vi "testSharedVariable.vi"() -> ()   [LabVIEW 2015]
uses:
  state.ctl
  MyToolsStatus.lvlib
panel:
  in  "Cluster":T1
  out "error out":errorcluster
  in  "stop":bool
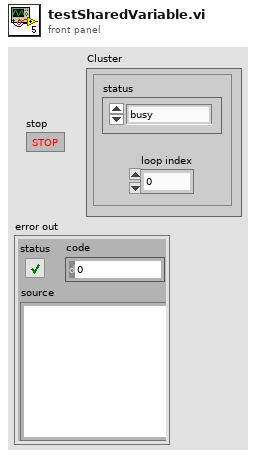
[diagram p1: front panel]
types:
  T1 = typedef "MyToolsStatus.lvlib/state.ctl" = cluster{"loop index":i32, "status":enum16{"busy", "ready", "error"}}
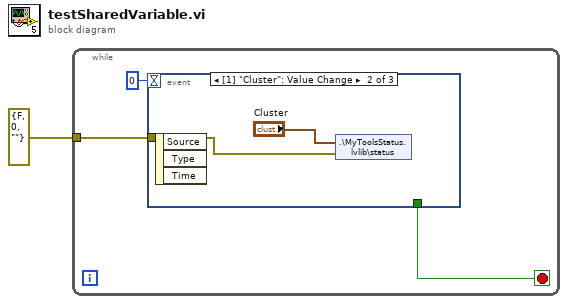
[diagram p0: block diagram]
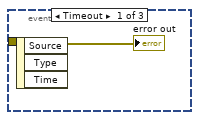
[diagram p2: hidden frame]
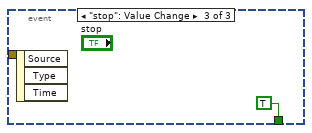
[diagram p3: hidden frame]
diagram:
  n1 = while {
    tunnel: errorcluster {"status"=FALSE, "code"=0, "source"=""} ("error in (no error)") -> [w4]
    stop <- w3 stop-if-true
    n2 = event shown="[1] \"Cluster\": Value Change" {
      selector: _ -> [_ _ _]
      dyn-events: _ -> [_ _ _]
      timeout: 0 -> [_ _ _]
      tunnel: w4 -> [w5 w7 _]
      tunnel: [_ _ TRUE] -> w3
      event Timeout {
        n3 = event-data() -> ()  [unwired: 1 in, 3 out]
        "error out" <- w5
      }
      event Value Change {
        n4 = event-data() -> ()  [unwired: 1 in, 3 out]
        n5 = shared-variable ".\\MyToolsStatus.lvlib\\status"("Cluster", error in=w7) -> ()  [unwired: 1 out]
      }
      event "stop": Value Change {
        n6 = event-data() -> ()  [unwired: 1 in, 3 out]
      }
    }
  }
